vi "IMU GUID Lookup.vi"() -> ()   [LabVIEW 2015, in "IMU Custom Device.lvlib"]
doc: "Use this Global VI to access the GUIDs assigned to the page resources of the Custom Device."
uses:
  IMU Custom Device.lvlib
panel:
  in  "Custom Device":string="cf94157c-4ce5-4e67-89d0-d741142684ed"
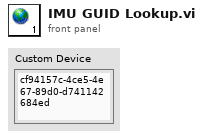
[diagram p1: front panel]
diagram:
